vi "3D Cartesian Coordinate Rotation (Euler) (Scalar).vi"(8 "Euler Angles":cluster{"phi":dbl, "theta":dbl, "psi":dbl}, 9 "z":dbl, 10 "y":dbl, 11 "x":dbl) -> (0 "error":i32, 1 "z out":dbl, 2 "y out":dbl, 3 "x out":dbl)   [LabVIEW 2010, in "NI_AALPro.lvlib"]
doc: "Rotates a three-dimensional Cartesian coordinate in the counterclockwise direction using the Euler angles method. Wire data to the <B>X</B> input to determine the polymorphic instance to use or manually select the instance."
uses:
  NI_AALPro.lvlib
  lvanlys.dll
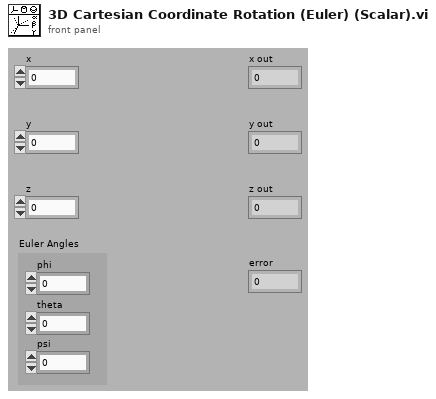
[diagram p1: front panel]
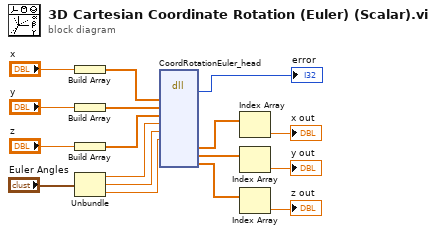
[diagram p0: block diagram]
diagram:
  n1 = Build Array("x") -> (w13:dbl[])
  n2 = Build Array("y") -> (w12:dbl[])
  n3 = Build Array("z") -> (w11:dbl[])
  n4 = Unbundle("Euler Angles") -> ("phi"=w8:dbl, "theta"=w7:dbl, "psi"=w6:dbl)
  n5 = dll-call lib="C:/Program Files/National Instruments/LabVIEW 2010/resource/lvanlys.*" fn="CoordRotationEuler_head"("X"=w13, "Y"=w12, "Z"=w11, "phi"=w8, "theta"=w7, "psi"=w6) -> (→"error":i32, "Xout"=w5:dbl[], "Yout"=w4:dbl[], "Zout"=w3:dbl[])  [unwired: 12 in, 2 out]
  n6 = Index Array(array=w5) -> (element=→"x out":dbl)  [unwired: 1 in]
  n7 = Index Array(array=w4) -> (element=→"y out":dbl)  [unwired: 1 in]
  n8 = Index Array(array=w3) -> (element=→"z out":dbl)  [unwired: 1 in]
